vi "INSERT_PRODUCT.vi"() -> ()   [LabVIEW 2020]
panel:
  in  "产品型号":u16(ring) caption="Enum 3"
  in  "插入壳体码":bool
  in  "插入传感器码":bool
  in  "设置状态":enum16{"", "OK", "NG"}(ring)
  out "当前状态":string
  in  "设备名称":u16(ring) caption="Enum 3" items=["", "芯轴分总成磨合台", "上管柱组件装配", "上管柱上转向轴合成", "滑移力检测", "芯轴分总成NVH", "上转向轴组件装配", "上下管柱总成装配", "滑移力复检", "最终性能试验台", "传感器对中台", "电机装配", "中间轴装配", "GP12（340）", "ECU装配", "激光打标机"]
  in  "追溯码":string
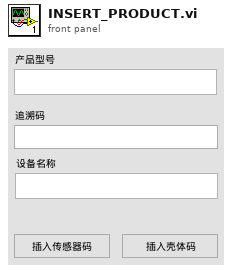
[diagram p1: front panel]
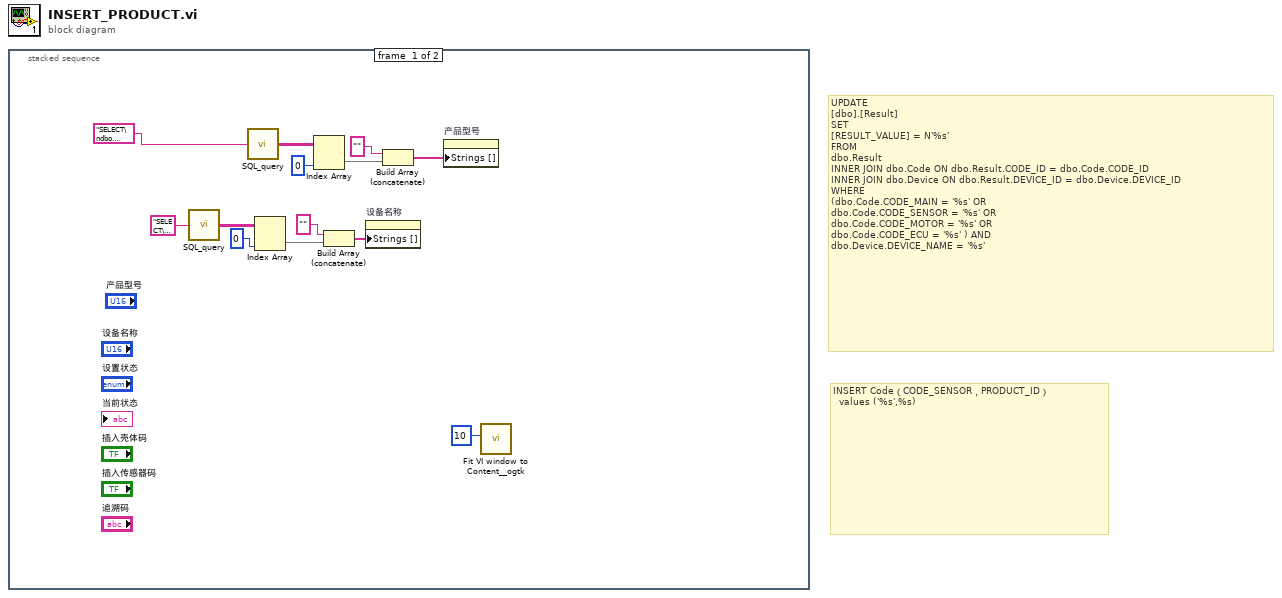
[diagram p0: block diagram]
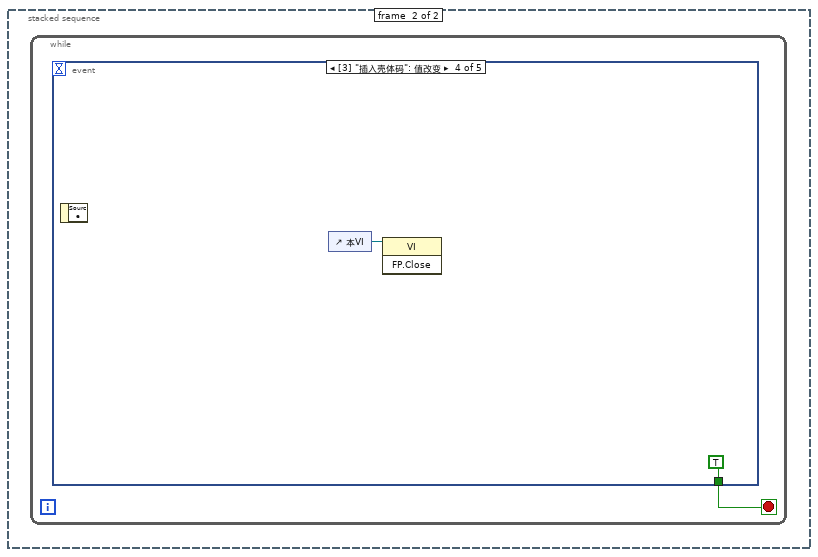
[diagram p2: hidden frame]
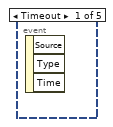
[diagram p3: hidden frame]
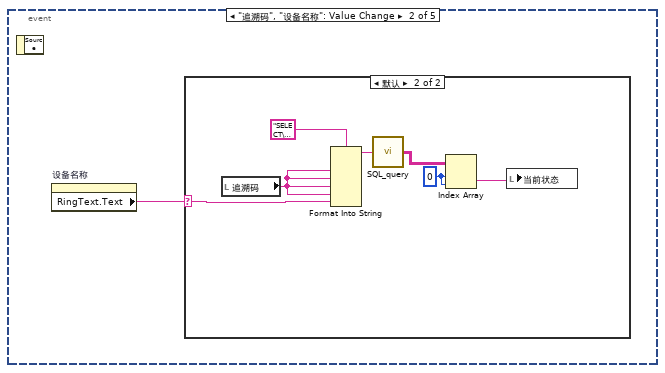
[diagram p4: hidden frame]
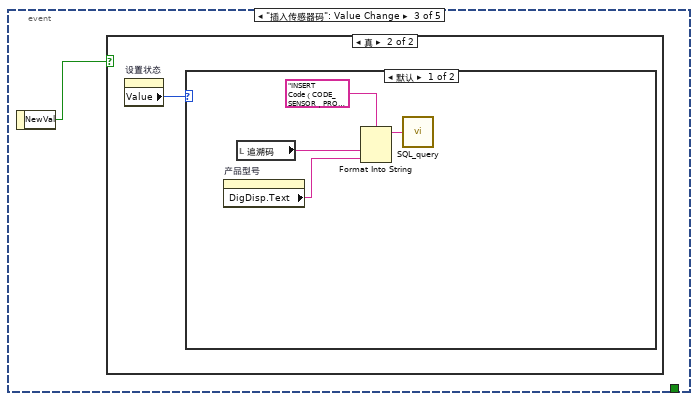
[diagram p6: hidden frame]
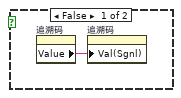
[diagram p7: hidden frame]
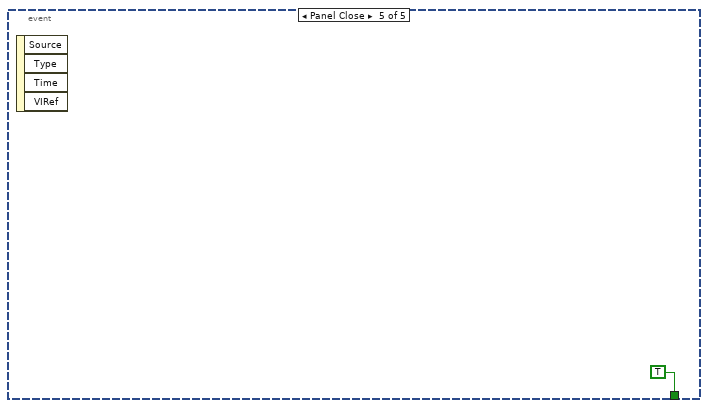
[diagram p9: hidden frame]
diagram:
  # "INSERT Code（CODE_SENSOR，PRODUCT_ID） \n  values ('%s',%s)"
  # "UPDATE \n[dbo].[Result] \nSET \n[RESULT_VALUE] = N'%s'\nFROM\ndbo.Result\nINNER JOIN dbo.Code ON dbo.Result.CODE_ID = dbo.Code.CODE_ID\nINNER JOIN dbo.Device ON dbo.Result.DEVICE_ID = dbo.Device.DEVICE_ID\nWHERE\n(dbo.Code.CODE_MAIN = '%s' OR\ndbo.Code.CODE_SENSOR = '%s' OR\ndbo.Code.CODE_MOTOR = '%s' OR\ndbo.Code.CODE_ECU = '%s' ) AND\ndbo.Device.DEVICE_NAME = '%s'"
  n1 = stacked-sequence {
    frame #0 {
      n2 = call "SQL_query.vi"("SQL query"="SELECT\ndbo.Device.DEVICE_NAME\n\nFROM\ndbo.Device\n") -> ("data"=w12:string[][])  [unwired: 3 in, 1 out]
      n3 = call "SQL_query.vi"("SQL query"="SELECT\ndbo.Product.PRODUCT_NAME\n\nFROM\ndbo.Product\n") -> ("data"=w6:string[][])  [unwired: 3 in, 1 out]
      n4 = Index Array(array=w12, index (col)=0 ("禁用的索引 (列)")) -> (element=w11:string[])  [unwired: 1 in]
      n5 = Index Array(array=w6, index (col)=0 ("禁用的索引 (列)")) -> (element=w4:string[])  [unwired: 1 in]
      n6 = Build Array (concatenate)("", w11) -> (w8:string[])
      n7 = property on="设备名称" class="Ring (严格)"("Strings []"=w8) -> ()  [unwired: 2 in, 2 out]
      n8 = Build Array (concatenate)("", w4) -> (w5:string[])
      n9 = property on="产品型号" class="Ring (严格)"("Strings []"=w5) -> ()  [unwired: 2 in, 2 out]
      n10 = call <userlib>:"Fit VI window to Content__ogtk.vi"("border spacing (2 px)"=10) -> ()  [unwired: 5 in, 2 out]
    }
    frame #1 {
      n11 = while {
        stop <- w14 stop-if-true
        n12 = event shown="[3] \"插入壳体码\": 值改变" {
          selector: _ -> [_ _ _ _ _]
          dyn-events: _ -> [_ _ _ _ _]
          timeout: _ -> [_ _ _ _ _]
          tunnel: [_ _ _ TRUE TRUE] -> w14
          event Timeout {
            n13 = event-data() -> ()  [unwired: 1 in, 3 out]
          }
          event "追溯码", "设备名称": Value Change {
            n14 = event-data() -> ()  [unwired: 1 in, 1 out]
            n15 = property on="设备名称" class="Ring (严格)"() -> ("RingText.Text"=w15:string)  [unwired: 2 in, 2 out]
            n16 = case shown="默认" w15 {
              selector: w15 -> [_ w20]
              frame "" {
              }
              frame Default {
                w18 = 0 ("索引 (行)")
                n17 = local read "追溯码"() -> (w22:string)
                n18 = Format Into String(format string="SELECT\n[dbo].[Result].[RESULT_VALUE] \nFROM\ndbo.Result\nINNER JOIN dbo.Code ON dbo.Result.CODE_ID = dbo.Code.CODE_ID\nINNER JOIN dbo.Device ON dbo.Result.DEVICE_ID = dbo.Device.DEVICE_ID\nWHERE\n(dbo.Code.CODE_MAIN = '%s' OR\ndbo.Code.CODE_SENSOR = '%s' OR\ndbo.Code.CODE_MOTOR = '%s' OR\ndbo.Code.CODE_ECU = '%s' ) AND\ndbo.Device.DEVICE_NAME = '%s'\n" ("格式字符串"), w22, w22, w22, w22, w20) -> (resulting string=w21:string)  [unwired: 2 in, 1 out]
                n19 = call "SQL_query.vi"("SQL query"=w21) -> ("data"=w19:string[][])  [unwired: 3 in, 1 out]
                n20 = Index Array(array=w19, index (row)=w18, index (col)=w18) -> (element=w17:string)
                n21 = local write "当前状态"(w17) -> ()
              }
            }
          }
          event "插入传感器码": Value Change {
            n22 = event-data() -> ("NewVal"=w23:bool)  [unwired: 1 in]
            n23 = case shown="真" w23 {
              frame False {
                n24 = property on="追溯码" class="Str"() -> ("Value"=w24:string)  [unwired: 2 in, 2 out]
                n25 = property on="追溯码" class="Str"("Val(Sgnl)"=w24) -> ()  [unwired: 2 in, 2 out]
              }
              frame True {
                n26 = property on="设置状态" class="Enum (严格)"() -> ("Value"=w25:enum16{"", "OK", "NG"})  [unwired: 2 in, 2 out]
                n27 = case shown="默认" w25 {
                  frame Default {
                    n28 = property on="产品型号" class="Ring (严格)"() -> ("DigDisp.Text"=w26:string)  [unwired: 2 in, 2 out]
                    n29 = local read "追溯码"() -> (w27:string)
                    n30 = Format Into String(format string="INSERT Code（CODE_SENSOR，PRODUCT_ID） \n  values ('%s',%s) " ("格式字符串"), w27, w26) -> (resulting string=w29:string)  [unwired: 2 in, 1 out]
                    n31 = call "SQL_query.vi"("SQL query"=w29) -> ()  [unwired: 3 in, 2 out]
                  }
                  frame "" {
                  }
                }
              }
            }
          }
          event "插入壳体码": Value Change {
            n32 = event-data() -> ()  [unwired: 1 in, 1 out]
            n33 = control-ref of="本VI"() -> (w30:refnum<vi>)
            n34 = invoke class="VI" method="FP.Close"(reference=w30) -> ()  [unwired: 2 in, 3 out]
          }
          event Panel Close {
            n35 = event-data() -> ()  [unwired: 1 in, 4 out]
          }
        }
      }
    }
  }
